vi "Note On.vi"(7 "Channel (1-16)":u8=1, 8 "error in (no error)":errorcluster, 9 "Velocity (0-127)":u8=80, 10 "MIDI Note Name":T1=enum."C4", 11 "midi out in":refnum<class "midi out.lvclass">) -> (0 "error out":errorcluster, 3 "midi out out":refnum<class "midi out.lvclass">)   [LabVIEW 2020, in "midi out.lvclass"]
uses:
  midi out.lvclass
  shared/midi note name.ctl
  shared/midi status byte.ctl
  midi out.lvclass/midi out.ctl
  shared/midi shared.lvlib
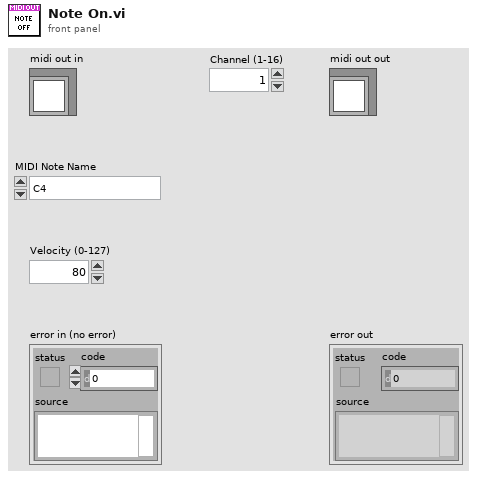
[diagram p1: front panel]
types:
  T1 = typedef "midi shared.lvlib/midi note name.ctl" = enum8{"C-1", "C#-1", "D-1", "D#-1", "E-1", "F-1", "F#-1", "G-1", "G#-1", "A-1", "A#-1", "B-1", "C0", "C#0", "D0", "D#0", "E0", "F0", "F#0", "G0", "G#0", "A0", "A#0", "B0", "C1", "C#1", "D1", "D#1", "E1", "F1", "F#1", "G1", "G#1", "A1", "A#1", "B1", "C2", "C#2", "D2", "D#2", "E2", "F2", "F#2", "G2", "G#2", "A2", "A#2", "B2", "C3", "C#3", "D3", "D#3", "E3", "F3", "F#3", "G3", "G#3", "A3", "A#3", "B3", "C4", "C#4", "D4", "D#4", "E4", "F4", "F#4", "G4", "G#4", "A4", "A#4", "B4", "C5", "C#5", "D5", "D#5", "E5", "F5", "F#5", "G5", "G#5", "A5", "A#5", "B5", "C6", "C#6", "D6", "D#6", "E6", "F6", "F#6", "G6", "G#6", "A6", "A#6", "B6", "C7", "C#7", "D7", "D#7", "E7", "F7", "F#7", "G7", "G#7", "A7", "A#7", "B7", "C8", "C#8", "D8", "D#8", "E8", "F8", "F#8", "G8", "G#8", "A8", "A#8", "B8", "C9", "C#9", "D9", "D#9", "E9", "F9", "F#9", "G9", "G#9", "A9", "A#9", "B9", "C10", "C#10", "D10", "D#10", "E10", "F10", "F#10", "G10"}
  T2 = typedef "midi shared.lvlib/midi status byte.ctl" = enum8{"Note Off Ch1", "Note Off Ch2", "Note Off Ch3", "Note Off Ch4", "Note Off Ch5", "Note Off Ch6", "Note Off Ch7", "Note Off Ch8", "Note Off Ch9", "Note Off Ch10", "Note Off Ch11", "Note Off Ch12", "Note Off Ch13", "Note Off Ch14", "Note Off Ch15", "Note Off Ch16", "Note On Ch1", "Note On Ch2", "Note On Ch3", "Note On Ch4", "Note On Ch5", "Note On Ch6", "Note On Ch7", "Note On Ch8", "Note On Ch9", "Note On Ch10", "Note On Ch11", "Note On Ch12", "Note On Ch13", "Note On Ch14", "Note On Ch15", "Note On Ch16", "Poly Aftertouch Ch1", "Poly Aftertouch Ch2", "Poly Aftertouch Ch3", "Poly Aftertouch Ch4", "Poly Aftertouch Ch5", "Poly Aftertouch Ch6", "Poly Aftertouch Ch7", "Poly Aftertouch Ch8", "Poly Aftertouch Ch9", "Poly Aftertouch Ch10", "Poly Aftertouch Ch11", "Poly Aftertouch Ch12", "Poly Aftertouch Ch13", "Poly Aftertouch Ch14", "Poly Aftertouch Ch15", "Poly Aftertouch Ch16", "Control Change Ch1", "Control Change Ch2", "Control Change Ch3", "Control Change Ch4", "Control Change Ch5", "Control Change Ch6", "Control Change Ch7", "Control Change Ch8", "Control Change Ch9", "Control Change Ch10", "Control Change Ch11", "Control Change Ch12", "Control Change Ch13", "Control Change Ch14", "Control Change Ch15", "Control Change Ch16", "Program Change Ch1", "Program Change Ch2", "Program Change Ch3", "Program Change Ch4", "Program Change Ch5", "Program Change Ch6", "Program Change Ch7", "Program Change Ch8", "Program Change Ch9", "Program Change Ch10", "Program Change Ch11", "Program Change Ch12", "Program Change Ch13", "Program Change Ch14", "Program Change Ch15", "Program Change Ch16", "Channel Aftertouch Ch1", "Channel Aftertouch Ch2", "Channel Aftertouch Ch3", "Channel Aftertouch Ch4", "Channel Aftertouch Ch5", "Channel Aftertouch Ch6", "Channel Aftertouch Ch7", "Channel Aftertouch Ch8", "Channel Aftertouch Ch9", "Channel Aftertouch Ch10", "Channel Aftertouch Ch11", "Channel Aftertouch Ch12", "Channel Aftertouch Ch13", "Channel Aftertouch Ch14", "Channel Aftertouch Ch15", "Channel Aftertouch Ch16", "Pitch Bend Ch1", "Pitch Bend Ch2", "Pitch Bend Ch3", "Pitch Bend Ch4", "Pitch Bend Ch5", "Pitch Bend Ch6", "Pitch Bend Ch7", "Pitch Bend Ch8", "Pitch Bend Ch9", "Pitch Bend Ch10", "Pitch Bend Ch11", "Pitch Bend Ch12", "Pitch Bend Ch13", "Pitch Bend Ch14", "Pitch Bend Ch15", "Pitch Bend Ch16", "System Exclusive Start", "MIDI Time Code Quarter Frame", "Song Position Pointer", "Song Select", "System Common Undefined F4", "System Common Undefined F5", "Tune Request", "System Exclusive End", "Timing Clock", "System Real-time Undefined F9", "Start", "Continue", "Stop", "System Real-time Undefined FD", "Active Sensing", "System Reset"}
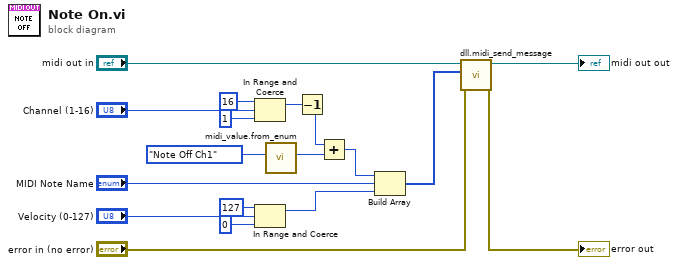
[diagram p0: block diagram]
diagram:
  n1 = In Range and Coerce(upper limit=u8 16, x="Channel (1-16)", lower limit=u8 1) -> (coerced(x)=w15:u8)  [unwired: 1 out]
  n2 = In Range and Coerce(upper limit=u8 127, x="Velocity (0-127)", lower limit=u8 0) -> (coerced(x)=w6:u8)  [unwired: 1 out]
  n3 = call "midi_value.from_enum.vi"("MIDI Status Byte"=midi_status_byte."Note Off Ch1") -> ("midi status value"=w13:u8)  [unwired: 10 in]
  n4 = Decrement(x=w15) -> (x-1=w12:u8)
  n5 = Add(x=w12, y=w13) -> (x+y=w8:u8)
  n6 = Build Array(w8, "MIDI Note Name", w6) -> (w5:u8[])
  n7 = call "dll.midi_send_message.vi"("error in (no error)"="error in (no error)", "message array (U8)"=w5, "midi out in"="midi out in") -> ("error out"=→"error out":errorcluster, "midi out"=→"midi out out":refnum<class "midi out.lvclass">)  [unwired: 7 in]
